vi "Calibration_user_input.vi"(4 "data mode":enum16{"Take new data point", "Refit Curve"}(ring), 6 "Mode":T5, 7 "Fixed n":bool, 8 "OK":T12, 9 "Sampling speeds":T6={"Samples /ch"=300, "Sampling Rate /ch (Hz)"=50.0} {"Sampling Rate /ch (Hz)" min=0 format="%.2f"; "Samples /ch" min=0 step=1}) -> (0 "Ch & Spans":T1[](array[typedef]) {"Ch No" min=0 max=7; "low limit (-10V)" min=-10 max=10 format="%.3f"; "high limit (10V)" min=-10 max=10 format="%.3f"}, 1 "Sampling speeds Output":T6={"Samples /ch"=300, "Sampling Rate /ch (Hz)"=50.0} {"Sampling Rate /ch (Hz)" min=0 format="%.2f"; "Samples /ch" min=0 step=1}, 2 "Fixed n out":bool, 3 "Temp (deg C)":dbl=21.0 format="%.1f", 5 "Abs Press (mbar)":dbl=1013.0 format="%.1f")   [LabVIEW 2013]
uses:
  Globals/Calib_global.vi
  Globals/Meas_global.vi
  Controls/Ref_Inst_type.ctl
  Controls/Setup.ctl
  Globals/LDA_meas_global_2.vi
  ADAM Client/Sub VIs/ADAM Controls/Channel_names.ctl
  Calib_mode.ctl
  Controls/Cal_Inst_type.ctl
  Controls/Inst_type.ctl
  Controls/PWA_Data.ctl
  Controls/ok_button.ctl
  Globals/LDA_meas_global_1.vi
  File/Setup_Filetype.ctl
  Controls/LDA_Setup.ctl
  Calib_setup.ctl
  Controls/Calibration.ctl
  Controls/TypeCalib.ctl
panel:
  in  "Acquisition Plug in":u16(ring) items=["ADAM_Server_Channels.vi", "Channels_and_Index.ctl", "DataTranslation.vi", "DT_With_Multiplexer.vi", "LDA_IP.vi", "NI-DAQmx.vi", "Simulate_kernal.vi"]
  in  "PWA Data":T2
  in  "Preston tube diammeter in mm":dbl min=0.0
  in  "Reference instrument Orig":T4={"high limit (10V)"=4.0, "low limit (-10V)"=0.0, "Ch No"=4, "Off ch no"=0, "Calib filename"=path "", "Ref Instrument type"=enum."Enter Value"} {"Off ch no" min=0 max=1; "Ch No" min=0 max=7; "low limit (-10V)" min=-10 max=10 format="%.1f"; "high limit (10V)" min=-10 max=10 format="%.1f"}
  out "Message":string
  in  "Ref Instrument type":T3
  out "Info":string
  out "XW Angle Calib Present?":bool
  out "XW Velocity Calib Present?":bool
  in  "Edit temp and Press":bool
  out "2nd ref instrument":T7={"2nd Ref type"=enum."LDA", "2nd inst present"=TRUE}
  in  "Ref vel for angle calib":T8={"high limit (10V)"=6.0, "low limit (-10V)"=0.0, "Ch No"=4, "Off ch no"=0, "Calib filename"=path "", "Ref Instrument type"=enum."LDA"} {"Off ch no" min=0 max=1; "Ch No" min=0 max=50; "low limit (-10V)" min=-10 max=10 format="%.1f"; "high limit (10V)" min=-10 max=10 format="%.1f"}
  out "Instrument type":T9=enum."Cross wire angle"
  in  "angle calib":T10(ring)
  in  "Reference instrument":T8={"high limit (10V)"=4.0, "low limit (-10V)"=0.0, "Ch No"=4, "Off ch no"=0, "Calib filename"=path "", "Ref Instrument type"=enum."Enter Value"} {"Off ch no" min=0 max=1; "Ch No" min=0 max=50; "low limit (-10V)" min=-10 max=10 format="%.1f"; "high limit (10V)" min=-10 max=10 format="%.1f"}
  in  "instrument to calibrate":T11=[{"high limit (10V)"=5.0, "low limit (-10V)"=3.0, "Ch No"=1, "Off ch no"=1, "DAQmx Channel"=""}, {"high limit (10V)"=5.0, "low limit (-10V)"=3.0, "Ch No"=2, "Off ch no"=1, "DAQmx Channel"=""}] {"Off ch no" min=0 max=1; "Ch No" min=0 max=1000; "low limit (-10V)" min=-10 max=10 format="%.3f"; "high limit (10V)" min=-10 max=10 format="%.3f"}
  in  "Instrument type":T9=enum."Pressure Transducer"
  out "Calib filename":path
  in  "Type":T1={"high limit (10V)"=4.0, "low limit (-10V)"=0.0, "Ch No"=4, "Var name"="LDA", "DAQmx Chan"=""} {"Ch No" min=0 max=7; "low limit (-10V)" min=-10 max=10 format="%.3f"; "high limit (10V)" min=-10 max=10 format="%.3f"}
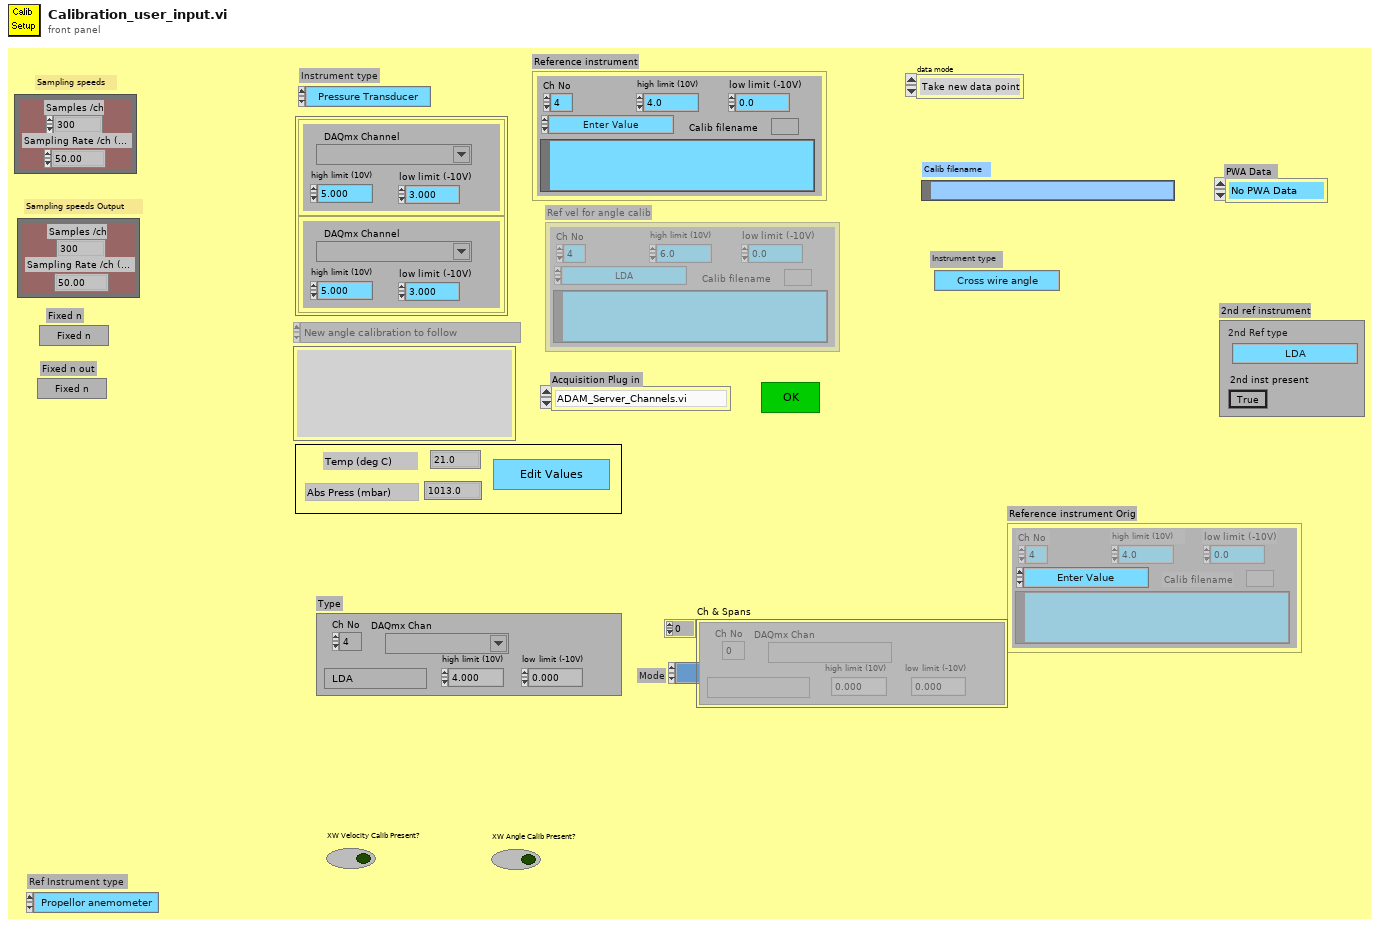
[diagram p1: front panel]
types:
  T1 = typedef "TypeCalib.ctl" = cluster{"high limit (10V)":sgl, "low limit (-10V)":sgl, "Ch No":i16, "Var name":string, "DAQmx Chan":tag}
  T2 = typedef "PWA_Data.ctl" = enum16{"No PWA Data", "One Ch PWA"}
  T3 = typedef "Ref_Inst_type.ctl" = enum16{"Propellor anemometer", "Pressure Transducer", "Raw voltage", "Pitot-static tube", "Preston tube", "Generic Linear", "Generic Polynomial", "Thermocouple", "LDA", "Enter Value", "ADAM Channel"}
  T4 = cluster{"high limit (10V)":sgl, "low limit (-10V)":sgl, "Ch No":i16, "Off ch no":i8, "Calib filename":path, "Ref Instrument type":T3}
  T5 = typedef "Calib_mode.ctl" = enum16{"Show Setup", "Take a New Calibration Point", "Refit Curve", "Setup Front Panel"}
  T6 = cluster{"Samples /ch":i32, "Sampling Rate /ch (Hz)":sgl}
  T7 = cluster{"2nd Ref type":T3, "2nd inst present":bool}
  T8 = typedef "Calib_setup.ctl" = cluster{"high limit (10V)":sgl, "low limit (-10V)":sgl, "Ch No":i16, "Off ch no":i8, "Calib filename":path, "Ref Instrument type":T3}
  T9 = typedef "Cal_Inst_type.ctl" = enum16{"Propeller anemometer", "Pressure Transducer", "Hot wire", "Cross wire velocity", "Cross wire angle", "Generic Linear", "Generic Polynomial", "Generic BackPoly", "Fast FID", "Thermocouple", "Cold wire", "Pulsed Wire"}
  T10 = enum16{"New angle calibration to follow", "Use the most recent angle calibration"}
  T11 = typedef "Calibration.ctl" = cluster{"high limit (10V)":sgl, "low limit (-10V)":sgl, "Ch No":i16, "Off ch no":i8, "DAQmx Channel":tag}[]
  T12 = typedef "ok_button.ctl" = bool
  T13 = typedef "Setup_Filetype.ctl" = enum16{"Measurement Setups", "Calibration Setups", "General", "Results File Plotter Setups", "Speed Calib Tweaks"}
  T14 = typedef "Inst_type.ctl" = enum16{"Propeller anemometer", "Raw voltage", "Pressure Transducer", "Pitot-static tube", "Preston tube", "Hot wire", "Cross wire 1", "Cross wire 2", "Generic Linear", "Generic Polynomial", "Generic BackPoly", "Fast FID", "Thermocouple", "Cold wire", "Pulsed Wire", "LDA Vel", "LDA Tran time", "LDA Arr time"}
  T15 = typedef "Channel_names.ctl" = enum16{"Active Only", "Active + Off", "All Channels"}
  T16 = typedef "LDA_Setup.ctl" = cluster{"dimensions":enum16{"1D", "2D"}, "Analogue Freq Multiplier":dbl}
  T17 = typedef "Setup.ctl" = enum16{"Run Program", "Show Setup", "Save Current Setup", "Setup Front Panel"}
  T18 = cluster{"high limit (10V)":sgl, "low limit (-10V)":sgl, "Ch No":i16, "Off ch no":i8, "DAQmx Channel":tag}
  T19 = typedef "BSA_Type.ctl" = enum16{"57N11", "BSA F60"}
  T20 = typedef "BSA_info_Cluster.ctl" = cluster{"GPIB Address":string, "No of Check Bytes":i32, "Extra Info":string, "COLOUR":u32, "Wavelength (nm)":dbl}
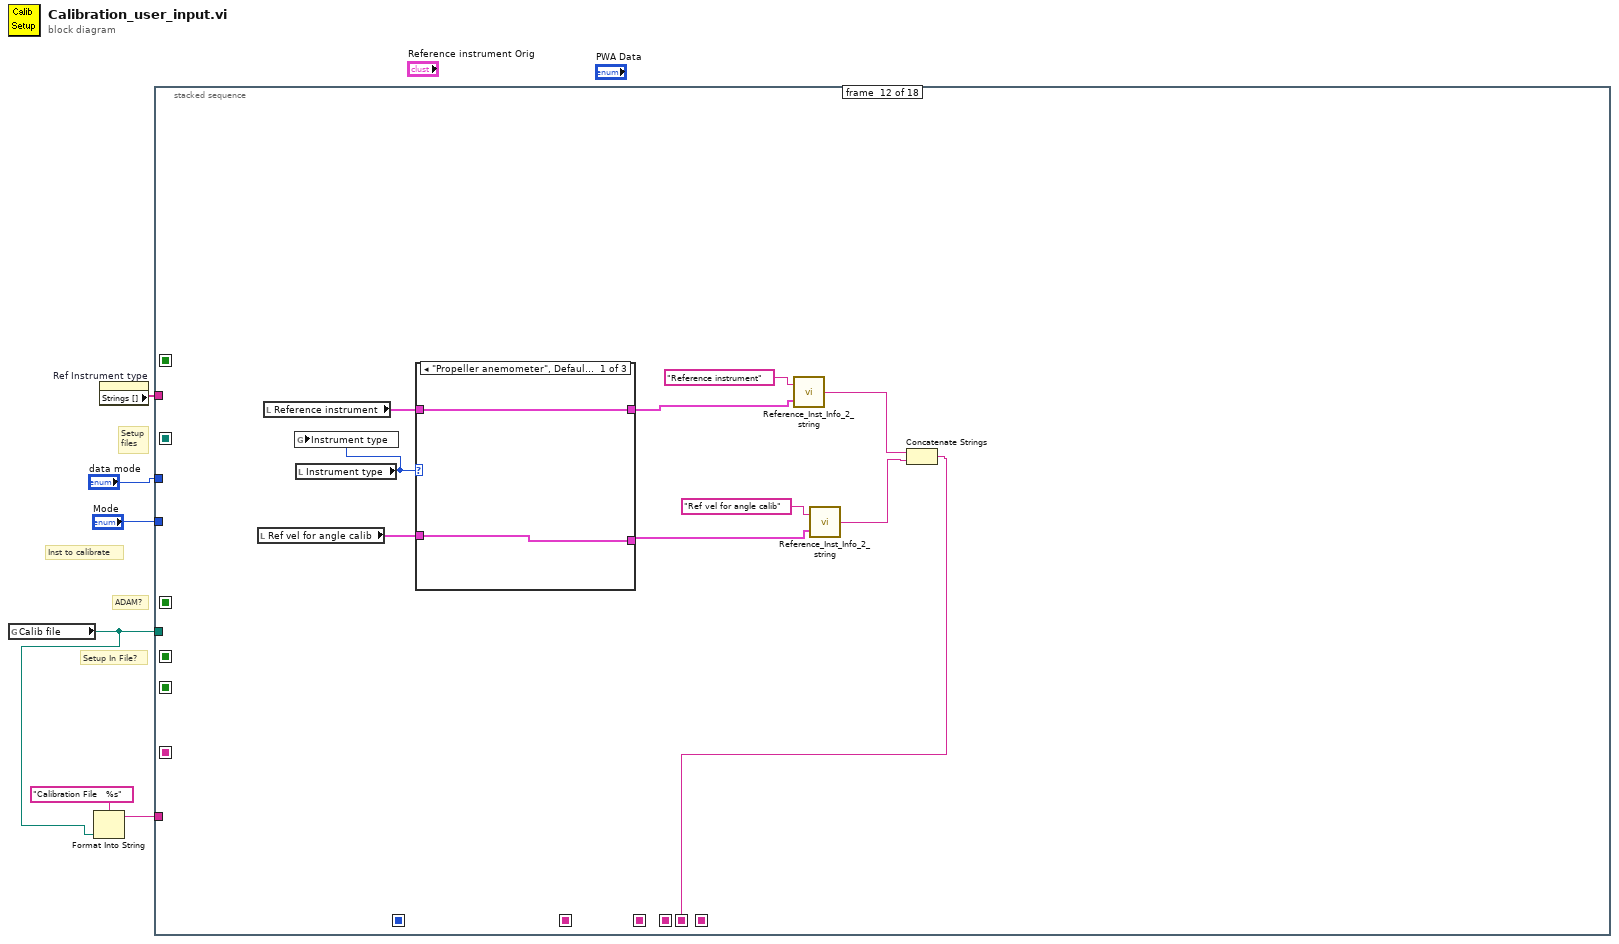
[diagram p0: block diagram]
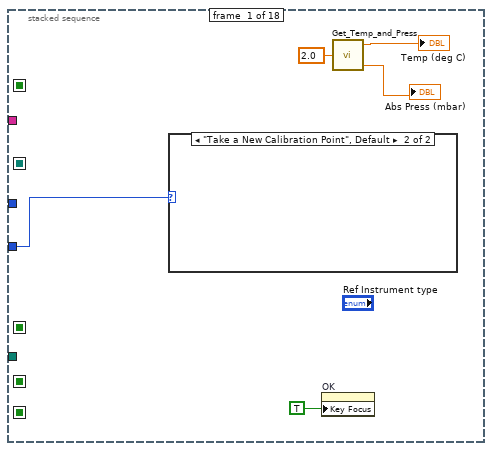
[diagram p2: hidden frame]
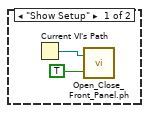
[diagram p3: hidden frame]
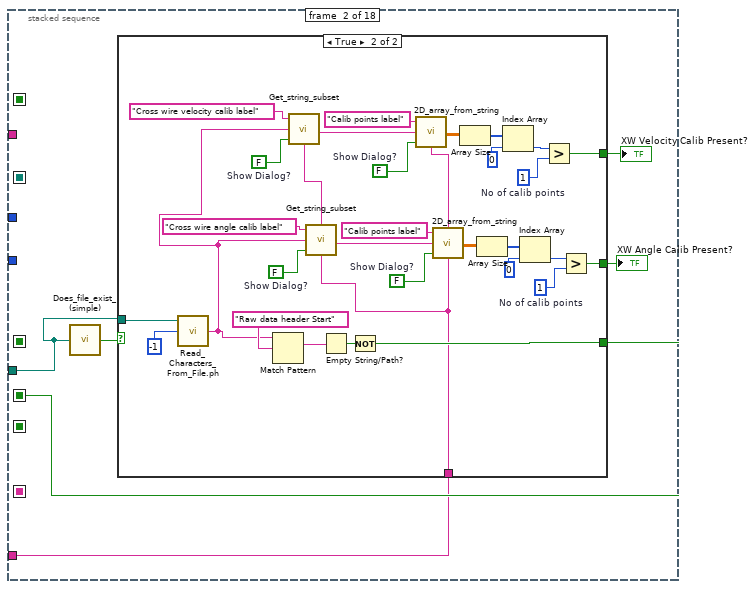
[diagram p4: hidden frame]
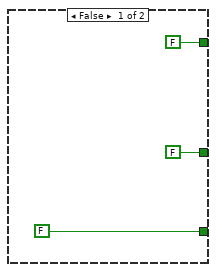
[diagram p5: hidden frame]
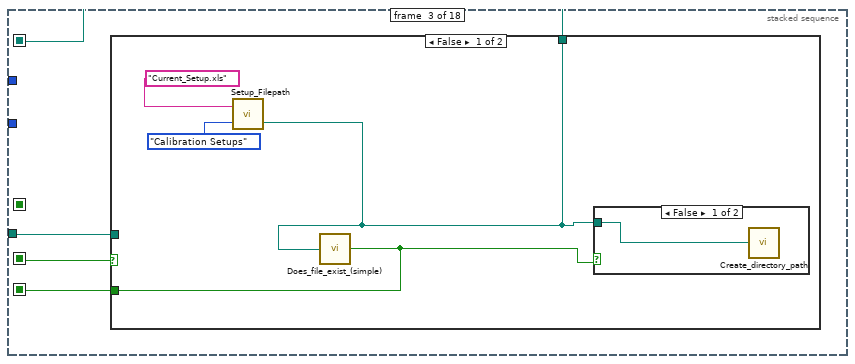
[diagram p6: hidden frame]
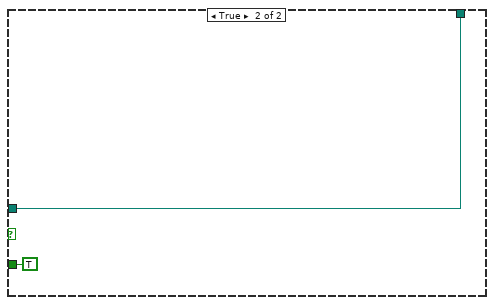
[diagram p8: hidden frame]
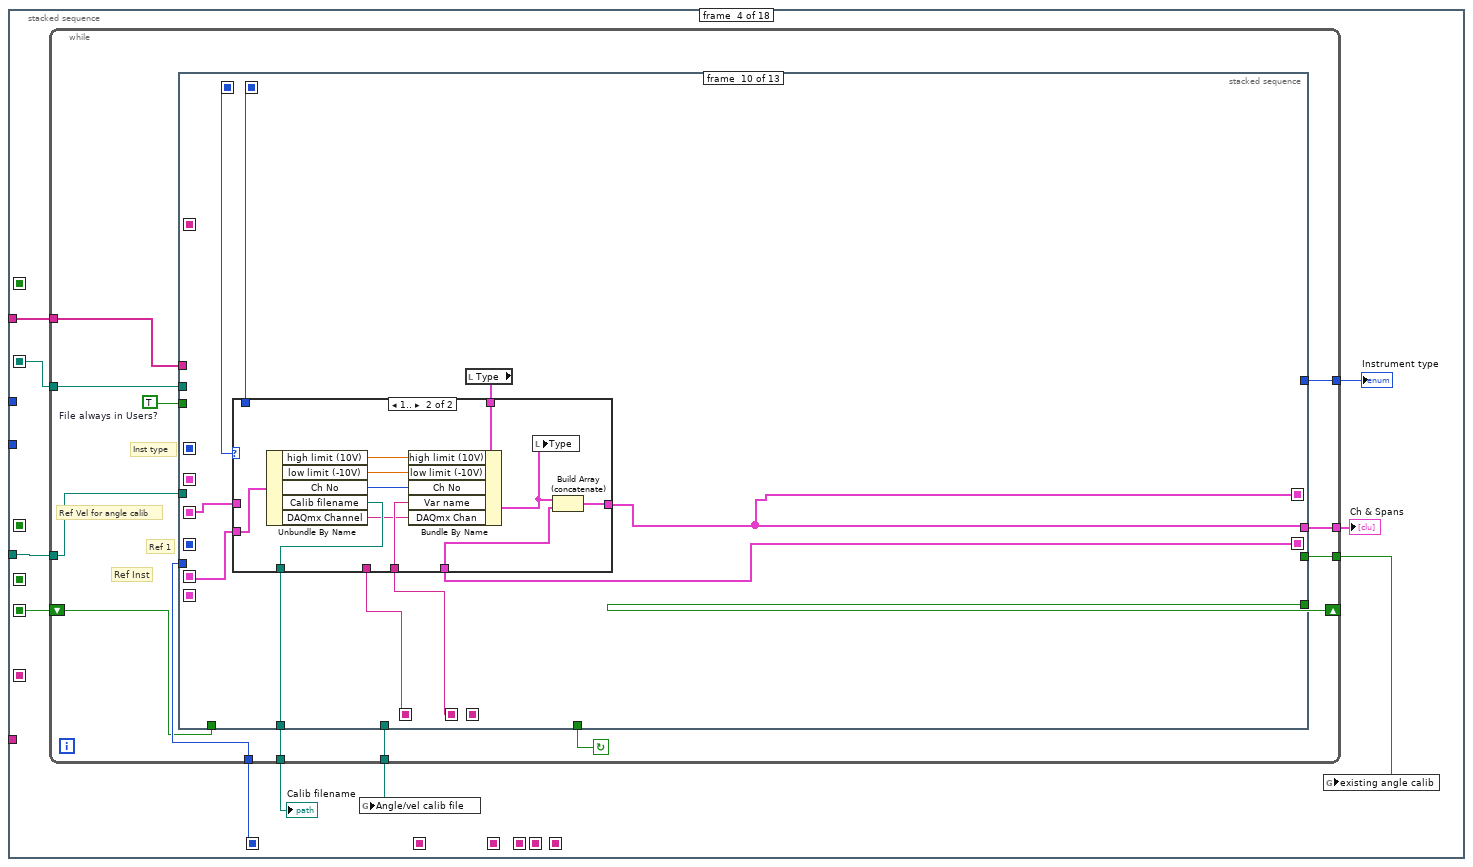
[diagram p9: hidden frame]
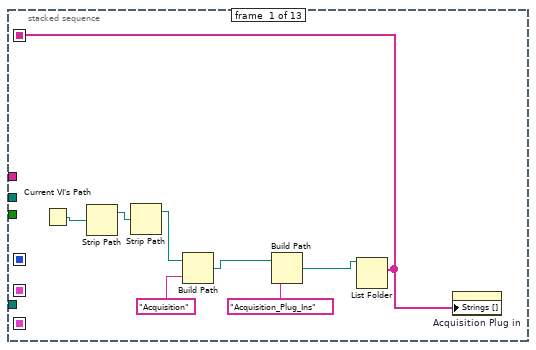
[diagram p10: hidden frame]
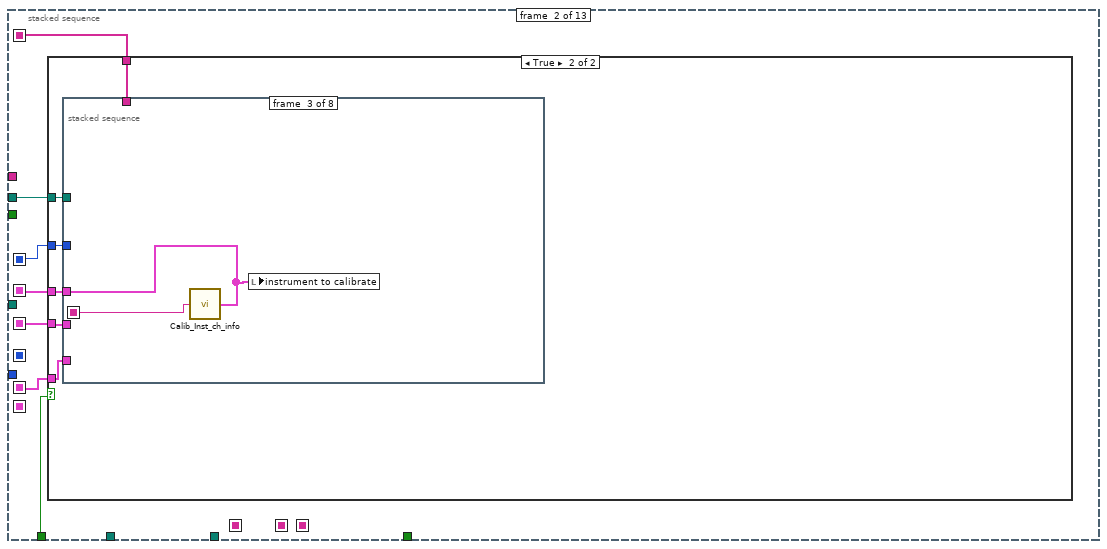
[diagram p11: hidden frame]
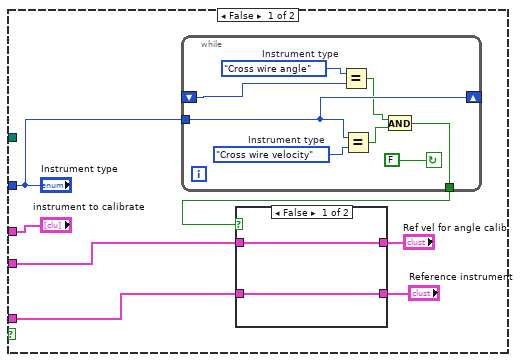
[diagram p12: hidden frame]
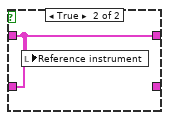
[diagram p13: hidden frame]
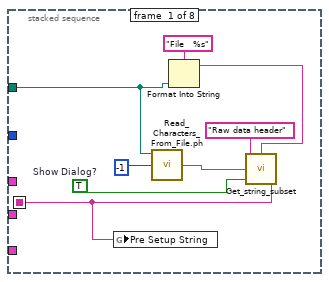
[diagram p14: hidden frame]
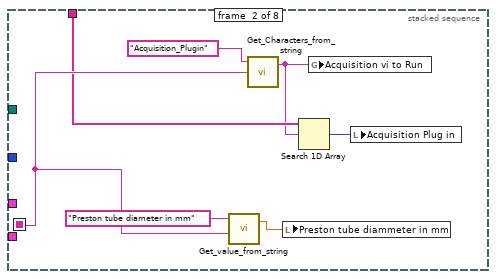
[diagram p15: hidden frame]
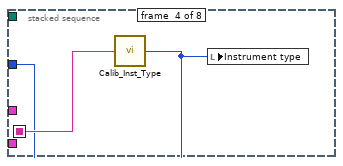
[diagram p16: hidden frame]
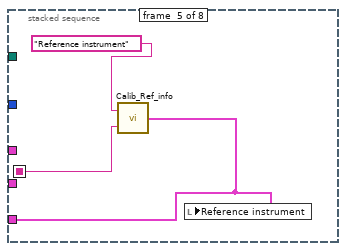
[diagram p17: hidden frame]
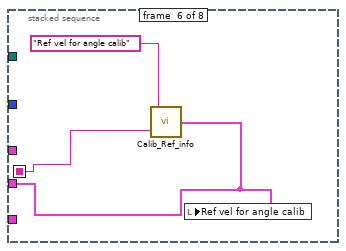
[diagram p18: hidden frame]
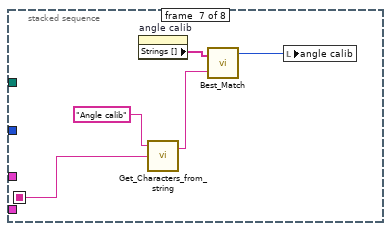
[diagram p19: hidden frame]
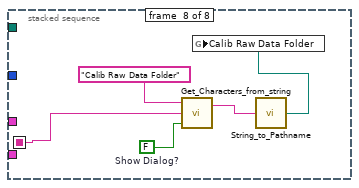
[diagram p20: hidden frame]
diagram:
  # "Inst to calibrate"
  # "Setup In File?"
  # "Setup\nfiles"
  # "ADAM?"
  n1 = global read "Calib_global.vi" "Calib file"() -> (w2:path)
  n2 = Format Into String(format string="Calibration File   %s", w2) -> (resulting string=w1:string)  [unwired: 2 in, 1 out]
  n3 = property on="Ref Instrument type" class="Enum (strict)"() -> ("Strings []"=w4:string[])  [unwired: 2 in, 2 out]
  n4 = stacked-sequence {
    seq-local: [_ _ w55 _ _ _ _ _ _ _ _ _ _ _ _ _ _ _] -> [_ _ _ w72 _ _ _ _ _ _ _ _ _ _ _ _ _ _]
    seq-local: [_ _ w56 _ _ _ _ _ _ _ _ _ _ _ _ _ _ _] -> [_ _ _ w70 _ _ _ _ _ _ _ _ _ _ _ _ _ _]
    seq-local: [_ _ _ w69 _ _ _ _ _ _ _ _ _ _ _ _ _ _] -> [_ _ _ _ _ _ _ w623 _ _ _ _ _ _ _ _ _ _]
    seq-local: [_ _ _ _ _ _ _ w624 _ _ _ _ _ _ _ _ _ _] -> [_ _ _ _ _ _ _ _ w641 _ _ _ _ _ _ _ _ _]
    seq-local: [_ _ _ _ _ _ _ _ w644 _ _ _ _ _ _ _ _ _] -> [_ _ _ _ _ _ _ _ _ _ _ _ _ _ w831 _ _ _]
    seq-local: [_ _ _ _ _ _ _ _ _ _ w733 _ _ _ _ _ _ _] -> [_ _ _ _ _ _ _ _ _ _ _ _ _ _ w830 _ w868 _]
    seq-local: [_ _ _ _ _ _ _ _ _ _ w730 _ _ _ _ _ _ _] -> [_ _ _ _ _ _ _ _ _ _ _ _ _ _ _ w837 _ _]
    seq-local: [_ w19 _ _ _ _ _ _ _ _ _ _ _ _ _ _ _ _] -> [_ _ w54 _ _ _ _ _ _ _ _ _ _ _ _ _ _ _]
    seq-local: [_ _ _ _ _ _ _ _ _ _ _ w745 _ _ _ _ _ _] -> [_ _ _ _ _ _ _ _ _ _ _ _ _ _ w823 _ _ _]
    seq-local: [_ _ _ _ _ _ _ _ _ _ _ _ _ w773 _ _ _ _] -> [_ _ _ _ _ _ _ _ _ _ _ _ _ _ w811 _ _ _]
    seq-local: [_ _ _ _ _ _ _ _ _ _ _ _ w752 _ _ _ _ _] -> [_ _ _ _ _ _ _ _ _ _ _ _ _ _ w807 _ w859 _]
    seq-local: [_ _ _ _ _ _ _ _ _ w679 _ _ _ _ _ _ _ _] -> [_ _ _ _ _ _ _ _ _ _ _ _ _ _ w806 _ _ _]
    tunnel: "Mode" -> [w7 _ _ _ w546 w564 _ _ w643 w692 _ _ w753 _ _ w839 _ w885]
    tunnel: "data mode" -> [_ _ _ _ w540 _ _ _ _ _ _ _ _ _ _ _ _ _]
    tunnel: w2 -> [_ w17 w53 w66 _ _ _ _ _ _ _ _ _ _ _ _ _ _]
    tunnel: w4 -> [_ _ _ w65 _ _ _ _ _ _ _ _ _ _ _ _ _ _]
    tunnel: w1 -> [_ w14 _ _ _ _ _ _ _ _ _ _ _ _ _ _ _ _]
    frame #0 {
      n5 = case shown="\"Take a New Calibration Point\", Default" w7 {
        frame "Show Setup" {
          n6 = Current VI's Path() -> (path=w13:path)
          n7 = call "Open_Close_Front_Panel.ph.vi"("Front Panel Window:Open"=TRUE, "VI path"=w13) -> ()  [unwired: 2 out]
        }
        frame "Take a New Calibration Point", Default {
        }
      }
      n8 = property on="OK" class="Bool"("Key Focus"=TRUE) -> ()  [unwired: 2 in, 2 out]
      n9 = call "Get_Temp_and_Press.vi"("Averaging time (mins)"=2.0) -> ("Abs Press (mbar)"=→"Abs Press (mbar)":dbl, "Temperature"=→"Temp (deg C)":dbl)  [unwired: 3 out]
    }
    frame #1 {
      n10 = call "Does_file_exist_(simple).vi"("Pathname"=w17) -> ("exists?"=w18:bool)
      n11 = case shown="True" w18 {
        tunnel: [FALSE w48] -> w19
        tunnel: w17 -> [_ w47]
        tunnel: [FALSE w25] -> w16
        tunnel: [FALSE w24] -> w15
        tunnel: w14 -> [_ w23]
        frame False {
        }
        frame True {
          w36 = 1  # No of calib points
          w30 = FALSE  # Show Dialog?
          w28 = FALSE  # Show Dialog?
          w37 = 1  # No of calib points
          w43 = FALSE  # Show Dialog?
          w45 = FALSE  # Show Dialog?
          n12 = call "Read_Characters_From_File.ph.vi"("file path (dialog if empty)"=w47, "number of characters (all:-1)"=-1) -> ("character string"=w26:string)  [unwired: 7 out]
          n13 = Match Pattern(string=w26, regular expression="Raw data header Start") -> (match substring=w50:string)  [unwired: 4 out]
          n14 = call "Get_string_subset.vi"("String Name"=w23, "Show Dialog?"=w28, "String to split"=w26, "File Label"="Cross wire velocity calib label") -> ("Output string"=w34:string)  [unwired: 1 out]
          n15 = call "Get_string_subset.vi"("String Name"=w23, "Show Dialog?"=w45, "String to split"=w26, "File Label"="Cross wire angle calib label") -> ("Output string"=w39:string)  [unwired: 1 out]
          n16 = Empty String/Path?(string/path=w50) -> (empty?=w49:bool)
          n17 = Not(x=w49) -> (.not. x?=w48:bool)
          n18 = call "2D_array_from_string.vi"("String Name"=w23, "Show Dialog?"=w30, "Input string"=w34, "Array title"="Calib points label") -> ("2D data array"=w31:dbl[][])
          n19 = call "2D_array_from_string.vi"("String Name"=w23, "Show Dialog?"=w43, "Input string"=w39, "Array title"="Calib points label") -> ("2D data array"=w42:dbl[][])
          n20 = Array Size(array=w31) -> (size(s)=w32:i32[])
          n21 = Array Size(array=w42) -> (size(s)=w41:i32[])
          n22 = Index Array(array=w32, index=0 ("Index")) -> (element=w35:i32)
          n23 = Index Array(array=w41, index=0 ("Index")) -> (element=w38:i32)
          n24 = Greater?(x=w35, y=w36) -> (0:w24:bool)
          n25 = Greater?(x=w38, y=w37) -> (0:w25:bool)
        }
      }
      "XW Velocity Calib Present?" <- w15
      "XW Angle Calib Present?" <- w16
    }
    frame #2 {
      n26 = case shown="False" w54 {
        tunnel: [w60 TRUE ("exists")] -> w56
        tunnel: [w57 w63] -> w55
        tunnel: w53 -> [_ w63]
        frame False {
          n27 = call "Setup_Filepath.vi"("Setup File Type"=Setup_Filetype."Calibration Setups", "Filename in"="Current_Setup.xls") -> ("Filename Out"=w57:path)  [unwired: 1 out]
          n28 = call "Does_file_exist_(simple).vi"("Pathname"=w57) -> ("exists?"=w60:bool)
          n29 = case shown="False" w60 {
            tunnel: w57 -> [w61 _]
            frame False {
              n30 = call "Create_directory_path.vi"("Path name"=w61) -> ()  [unwired: 1 in, 2 out]
            }
            frame True {
            }
          }
        }
        frame True {
        }
      }
    }
    frame #3 {
      n31 = while {
        tunnel: w65 -> [w77]
        shift-left: w70 -> [w80]
        shift-right: [w79] -> _
        tunnel: [w81] -> w71
        tunnel: w72 -> [w82]
        tunnel: [w83] -> w68
        tunnel: [w84] -> w64
        tunnel: [w85] -> w69
        tunnel: [w86] -> w73
        tunnel: [w75] -> w67
        tunnel: w66 -> [w74]
        stop <- w78 continue-if-true
        w76 = TRUE  # File always in Users?
        # "Ref 1"
        # "Ref Inst"
        # "Ref Vel for angle calib"
        # "Inst type"
        n32 = stacked-sequence {
          seq-local: [_ _ w166 _ _ _ _ _ _ _ _ _ _] -> [_ _ _ _ _ w290 _ _ _ _ _ _ _]
          seq-local: [_ _ w170 _ _ _ _ _ _ _ _ _ _] -> [_ _ _ _ _ _ _ _ w441 _ _ _ _]
          seq-local: [_ _ _ _ _ w284 _ _ _ _ _ _ _] -> [_ _ _ _ _ _ _ _ _ w459 _ _ _]
          seq-local: [_ _ w165 _ _ _ _ _ _ _ _ _ _] -> [_ _ _ _ _ _ _ _ _ w457 _ _ _]
          seq-local: [_ _ _ _ _ _ _ _ w440 _ _ _ _] -> [_ _ _ _ _ _ _ _ _ w458 _ _ _]
          seq-local: [_ _ _ _ _ _ _ w362 _ _ _ _ _] -> [_ _ _ _ _ _ _ _ _ w454 _ _ _]
          seq-local: [_ _ _ _ _ _ w358 _ _ _ _ _ _] -> [_ _ _ _ _ _ _ _ _ w453 _ _ _]
          seq-local: [_ w99 _ _ _ _ _ _ _ _ _ _ _] -> [_ _ w168 w201 w214 _ _ w363 _ _ _ _ _]
          seq-local: [_ w98 _ _ _ _ _ _ _ _ _ _ _] -> [_ _ _ w200 _ _ _ _ _ _ _ _ _]
          seq-local: [_ w97 _ _ _ _ _ _ _ _ _ _ _] -> [_ _ _ _ _ _ w360 w364 _ w452 _ _ _]
          seq-local: [_ w96 _ _ _ _ _ _ _ _ _ _ _] -> [_ _ w167 _ _ _ _ _ _ w451 _ _ w539]
          seq-local: [_ _ _ _ _ _ _ _ _ w450 _ _ _] -> [_ _ _ _ _ _ _ _ _ _ _ w498 _]
          seq-local: [_ _ _ w196 _ _ _ _ _ _ _ _ _] -> [_ _ _ _ _ _ _ _ w439 _ _ _ _]
          seq-local: [w87 _ _ _ _ _ _ _ _ _ _ _ _] -> [_ w95 _ _ _ _ _ _ _ _ _ _ _]
          tunnel: [_ _ _ _ _ _ _ _ _ w456 _ _ _] -> w86
          tunnel: [_ _ w166 _ _ _ _ _ _ _ _ _ _] -> w85
          tunnel: [_ _ _ _ _ _ _ _ _ w450 _ _ _] -> w84
          tunnel: [_ _ _ _ w219 _ _ _ _ _ _ _ _] -> w83
          tunnel: w82 -> [_ w101 _ _ _ _ _ _ _ _ _ _ _]
          tunnel: [_ _ w168 _ _ _ _ _ _ _ _ _ _] -> w81
          tunnel: w80 -> [_ w100 _ _ _ _ _ _ _ _ _ _ _]
          tunnel: [_ _ _ _ _ _ _ _ _ _ _ FALSE _] -> w79
          tunnel: [_ _ _ _ _ _ _ _ _ _ _ w496 _] -> w78
          tunnel: w77 -> [_ _ w164 _ _ _ w357 _ _ _ _ _ _]
          tunnel: w76 -> [_ _ _ _ _ _ _ _ _ _ _ _ _]
          tunnel: [_ _ _ _ w218 _ _ _ _ _ _ _ _] -> w75
          tunnel: w74 -> [_ _ _ _ w220 _ _ _ _ _ _ _ _]
          frame #0 {
            n33 = Current VI's Path() -> (path=w90:path)
            n34 = Strip Path(path=w90) -> (stripped path=w89:path)  [unwired: 1 out]
            n35 = Strip Path(path=w89) -> (stripped path=w88:path)  [unwired: 1 out]
            n36 = Build Path(base path=w88, name or relative path="Acquisition") -> (appended path=w93:path)
            n37 = Build Path(base path=w93, name or relative path="Acquisition_Plug_Ins") -> (appended path=w94:path)
            n38 = List Folder(path=w94) -> (filenames=w87:string[])  [unwired: 3 in, 3 out]
            n39 = property on="Acquisition Plug in" class="Ring (strict)"("Strings []"=w87) -> ()  [unwired: 2 in, 2 out]
          }
          frame #1 {
            n40 = case shown="True" w100 {
              tunnel: w101 -> [_ w125]
              tunnel: ["Instrument type" w123] -> w99
              tunnel: ["instrument to calibrate" w124] -> w98
              tunnel: [w103 w121] -> w97
              tunnel: [w105 w122] -> w96
              tunnel: w95 -> [_ w120]
              frame False {
                n41 = while {
                  shift-right: [w117] -> _
                  shift-left: _ -> [w115]
                  tunnel: "Instrument type" -> [w117]
                  tunnel: [w112] -> w106
                  stop <- FALSE continue-if-true
                  w116 = Cal_Inst_type."Cross wire angle"  # Instrument type
                  w118 = Cal_Inst_type."Cross wire velocity"  # Instrument type
                  n42 = Equal?(x=w116, y=w115) -> (x = y?=w113:bool)
                  n43 = Equal?(x=w117, y=w118) -> (x = y?=w114:bool)
                  n44 = And(x=w113, y=w114) -> (x .and. y?=w112:bool)
                }
                n45 = case shown="False" w106 {
                  tunnel: [w110 w111] -> w105
                  tunnel: "Reference instrument" -> [w110 _]
                  tunnel: [w109 w111] -> w103
                  tunnel: "Ref vel for angle calib" -> [w109 w111]
                  frame False {
                  }
                  frame True {
                    n46 = local write "Reference instrument"(w111) -> ()
                  }
                }
              }
              frame True {
                n47 = stacked-sequence {
                  seq-local: [w130 _ _ _ _ _ _ _] -> [_ w137 w142 w144 w146 w149 w153 w158]
                  tunnel: w125 -> [w127 _ _ _ _ _ _ _]
                  tunnel: [_ _ w141 _ _ _ _ _] -> w124
                  tunnel: [_ _ _ w143 _ _ _ _] -> w123
                  tunnel: [_ _ _ _ w145 _ _ _] -> w122
                  tunnel: [_ _ _ _ _ w148 _ _] -> w121
                  tunnel: w120 -> [_ w136 _ _ _ _ _ _]
                  frame #0 {
                    w129 = TRUE  # Show Dialog?
                    n48 = call "Read_Characters_From_File.ph.vi"("file path (dialog if empty)"=w127, "number of characters (all:-1)"=-1) -> ("character string"=w133:string)  [unwired: 7 out]
                    n49 = Format Into String(format string="File   %s", w127) -> (resulting string=w126:string)  [unwired: 2 in, 1 out]
                    n50 = call "Get_string_subset.vi"("String Name"=w126, "Show Dialog?"=w129, "String to split"=w133, "File Label"="Raw data header") -> ("Output string"=w130:string)  [unwired: 1 out]
                    n51 = global write "Calib_global.vi" "Pre Setup String"(w130) -> ()
                  }
                  frame #1 {
                    n52 = call "Get_value_from_string.vi"("Input string"=w137, "Variable name"="Preston tube diameter in mm") -> ("Value"=w139:dbl)  [unwired: 1 in, 1 out]
                    n53 = call "Get_Characters_from_string.vi"("Input string"=w137, "Variable name"="Acquisition_Plugin") -> ("Value"=w135:string)  [unwired: 1 in, 1 out]
                    n54 = local write "Preston tube diammeter in mm"(w139) -> ()
                    n55 = Search 1D Array(1D array=w136, element=w135) -> (index of element=w134:i32)  [unwired: 1 out]
                    n56 = global write "Meas_global.vi" "Acquisition vi to Run"(w135) -> ()
                    n57 = local write "Acquisition Plug in"(w134) -> ()
                  }
                  frame #2 {
                    n58 = call "Calib_Inst_ch_info.vi"("Input string"=w142) -> ("instrument to calibrate (new)"=w141:T11)
                    n59 = local write "instrument to calibrate"(w141) -> ()
                  }
                  frame #3 {
                    n60 = call "Calib_Inst_Type.vi"("Input string"=w144) -> ("Instrument type"=w143:T9)
                    n61 = local write "Instrument type"(w143) -> ()
                  }
                  frame #4 {
                    n62 = call "Calib_Ref_info.vi"("Input string"=w146, "Reference Name"="Reference instrument") -> ("Reference instrument"=w145:T8)
                    n63 = local write "Reference instrument"(w145) -> ()
                  }
                  frame #5 {
                    n64 = call "Calib_Ref_info.vi"("Input string"=w149, "Reference Name"="Ref vel for angle calib") -> ("Reference instrument"=w148:T8)
                    n65 = local write "Ref vel for angle calib"(w148) -> ()
                  }
                  frame #6 {
                    n66 = property on="angle calib" class="Enum (strict)"() -> ("Strings []"=w155:string[])  [unwired: 2 in, 2 out]
                    n67 = call "Get_Characters_from_string.vi"("Input string"=w153, "Variable name"="Angle calib") -> ("Value"=w152:string)  [unwired: 1 in, 1 out]
                    n68 = call "Best_Match.vi"("Input String"=w152, "String Options"=w155) -> ("index of element"=w151:i32)  [unwired: 1 out]
                    n69 = local write "angle calib"(w151) -> ()
                  }
                  frame #7 {
                    w159 = FALSE  # Show Dialog?
                    n70 = call "Get_Characters_from_string.vi"("Show Dialog?"=w159, "Input string"=w158, "Variable name"="Calib Raw Data Folder") -> ("Value"=w157:string)  [unwired: 1 out]
                    n71 = call "String_to_Pathname.vi"("Input String"=w157) -> ("path"=w156:path)
                    n72 = global write "Calib_global.vi" "Calib Raw Data Folder"(w156) -> ()
                  }
                }
              }
            }
          }
          frame #2 {
            # "#optimation Added 11/1/13"
            n73 = Unbundle By Name(w167) -> ("Ref Instrument type"=w169:T3)
            n74 = case shown="\"Cross wire angle\"" w168 {
              tunnel: [w181 w189 w194] -> w170
              tunnel: w169 -> [w179 w183 w193]
              tunnel: [w179 w186 w193] -> w166
              tunnel: w167 -> [_ w187 _]
              frame "Cross wire velocity" {
                n75 = Build Array("Raw voltage", "Raw voltage") -> (w181:string[])
              }
              frame "Cross wire angle" {
                n76 = case shown="\"ADAM Channel\"" w183 {
                  tunnel: [w190 w191 Ref_Inst_type."Enter Value" ("Ref Instrument type")] -> w186
                  tunnel: w183 -> [w190 w191 _]
                  frame "Enter Value" {
                  }
                  frame "ADAM Channel" {
                  }
                  frame "LDA", Default {
                  }
                }
                n77 = Bundle By Name(cluster=w187, "Ref Instrument type"=w186) -> (w188:T8)
                n78 = local write "Reference instrument"(w188) -> ()
                n79 = Build Array("Raw voltage", "Raw voltage") -> (w189:string[])
              }
              frame "Generic Linear", Default {
                n80 = Build Array("Raw voltage") -> (w194:string[])
              }
            }
            n81 = Index Array(array=w164, index=w166) -> (element=w165:string)
            n82 = property on="Acquisition Plug in" class="Ring (strict)"() -> ("Strings []"=w163:string[])  [unwired: 2 in, 2 out]
            n83 = Index Array(array=w163, index="Acquisition Plug in") -> (element=w161:string)
            n84 = case shown="\"NI-DAQmx.vi\"" w161 {
              frame "False", Default {
                (unwired) FALSE ("Visible")
                (unwired) FALSE ("Visible")
                n85 = property on="DAQmx Channel" class="DAQmxName"("Visible"=FALSE) -> ()  [unwired: 2 in, 2 out]
                n86 = property on="Ch No" class="DigNum (strict)"("Visible"=TRUE) -> ()  [unwired: 2 in, 2 out]
                n87 = property on="Ch No" class="DigNum (strict)"("Visible"=TRUE) -> ()  [unwired: 2 in, 2 out]
                n88 = property on="Ch No" class="DigNum (strict)"("Visible"=TRUE) -> ()  [unwired: 2 in, 2 out]
              }
              frame "NI-DAQmx.vi" {
                (unwired) TRUE ("Visible")
                (unwired) TRUE ("Visible")
                n89 = property on="DAQmx Channel" class="DAQmxName"("Visible"=TRUE) -> ()  [unwired: 2 in, 2 out]
                n90 = property on="Ch No" class="DigNum (strict)"("Visible"=FALSE) -> ()  [unwired: 2 in, 2 out]
                n91 = property on="Ch No" class="DigNum (strict)"("Visible"=FALSE) -> ()  [unwired: 2 in, 2 out]
                n92 = property on="Ch No" class="DigNum (strict)"("Visible"=FALSE) -> ()  [unwired: 2 in, 2 out]
              }
            }
            n93 = global write "Meas_global.vi" "Acquisition vi to Run"(w161) -> ()
          }
          frame #3 {
            n94 = Array Size(array=w200) -> (size(s)=w199:i32)
            n95 = case shown="\"Cross wire angle\"" w201 {
              tunnel: [2 2 1 0] -> w198
              frame "Cross wire velocity" {
              }
              frame "Cross wire angle" {
              }
              frame "Generic Linear", Default {
              }
              frame "Pulsed Wire" {
              }
            }
            n96 = Equal?(x=w198, y=w199) -> (x = y?=w197:bool)
            n97 = case shown="False" w197 {
              tunnel: w198 -> [w207 _]
              tunnel: w200 -> [w203 w209]
              tunnel: [w202 w209] -> w196
              frame False {
                n98 = Index Array(array=w203, index=0) -> (element=w204:T18)
                n99 = Build Array (concatenate)(w203, w204) -> (w206:T11)
                n100 = for {
                  N: w207 -> [_]
                  tunnel: w206 -> [w208] mode=indexing
                  tunnel: [w208] -> w202 mode=indexing
                }
                n101 = local write "instrument to calibrate"(w202) -> ()
              }
              frame True {
              }
            }
          }
          frame #4 {
            n102 = case shown="\"Cross wire angle\"" w214 {
              tunnel: w220 -> [_ w231 w253]
              tunnel: [path "" w232 w254] -> w219
              tunnel: [FALSE w230 w252] -> w218
              tunnel: [w221 w226 w248] -> w217
              tunnel: [w223 w229 w251] -> w216
              tunnel: ["" w228 w249] -> w215
              tunnel: w214 -> [_ w227 w250]
              frame "Propeller anemometer", Default {
                w221 = u8 2  # Disabled
                w223 = u8 2  # Disabled
              }
              frame "Cross wire angle" {
                w226 = u8 0  # Disabled
                w229 = u8 2  # Disabled
                n103 = local read "XW Velocity Calib Present?"() -> (w233:bool)
                n104 = case shown="False" w233 {
                  tunnel: [w237 w247] -> w232
                  tunnel: w231 -> [_ w247]
                  tunnel: [TRUE TRUE] -> w230
                  tunnel: [w235 w245] -> w228
                  tunnel: w227 -> [w234 _]
                  frame False {
                    w241 = 0  # index
                    n105 = local read "instrument to calibrate"() -> (w242:T11)
                    n106 = Index Array(array=w242, index=w241) -> (element=w240:T18)
                    n107 = Unbundle By Name(w240) -> ("Ch No"=w238:i16)
                    n108 = call "XW_file_info.vi"("Instrument type"=w234, "Ch No"=w238) -> ("Filename"=w237:path, "resulting string"=w235:string, "File Exists?"=w236:bool)
                    n109 = case shown="False" w236 {
                      frame False {
                        w243 = Cal_Inst_type."Cross wire velocity"  # Instrument type
                        w244 = "You need to do a velocity calibration before you can do the angle calibration"  # message
                        n110 = local write "Instrument type"(w243) -> ()
                        n111 = One Button Dialog(message=w244) -> ()  [unwired: 2 out]
                      }
                      frame True {
                      }
                    }
                  }
                  frame True {
                    w245 = "Will use the velocity Calibration info already in the Calibration file. "  # resulting string
                  }
                }
              }
              frame "Cross wire velocity" {
                w248 = u8 2  # Disabled
                n112 = local read "XW Angle Calib Present?"() -> (w255:bool)
                n113 = case shown="False" w255 {
                  tunnel: [w264 w283] -> w254
                  tunnel: w253 -> [_ w283]
                  tunnel: [TRUE FALSE] -> _
                  tunnel: [w263 TRUE] -> w252
                  tunnel: [w262 w280] -> w251
                  tunnel: w250 -> [w260 _]
                  tunnel: [w257 w279] -> w249
                  frame False {
                    w268 = 0  # index
                    n114 = local read "instrument to calibrate"() -> (w269:T11)
                    n115 = Index Array(array=w269, index=w268) -> (element=w267:T18)
                    n116 = Unbundle By Name(w267) -> ("Ch No"=w261:i16)
                    n117 = call "XW_file_info.vi"("Instrument type"=w260, "Ch No"=w261) -> ("Filename"=w259:path, "resulting string"=w256:string, "File Exists?"=w258:bool)
                    n118 = case shown="\"New angle calibration to follow\"" "angle calib" {
                      tunnel: [path "" w275] -> w264
                      tunnel: w259 -> [_ w275]
                      tunnel: [FALSE TRUE] -> w263
                      tunnel: ["This XW velocity Calibration MUST be followed by an angle calibration, before XW measurements can be made." w273] -> w257
                      tunnel: w256 -> [_ w273]
                      frame "New angle calibration to follow" {
                      }
                      frame "Use the most recent angle calibration" {
                      }
                    }
                    n119 = case shown="False" w258 {
                      tunnel: [w276 w278] -> w262
                      frame False {
                        w276 = u8 2  # Disabled
                        w277 = T10."New angle calibration to follow"  # angle calib
                        n120 = local write "angle calib"(w277) -> ()
                      }
                      frame True {
                        w278 = u8 0  # Disabled
                      }
                    }
                  }
                  frame True {
                    w279 = "Will use the angle Calibration info already in the Calibration file. "  # resulting string
                    w280 = u8 0  # Disabled
                  }
                }
              }
            }
            "Info" <- w215
            n121 = property on="Ref vel for angle calib" class="Clust (strict)"("Disabled"=w217) -> ()  [unwired: 2 in, 2 out]
            n122 = property on="angle calib" class="Enum (strict)"("Disabled"=w216) -> ()  [unwired: 2 in, 2 out]
          }
          frame #5 {
            n123 = case shown="\"Enter Value\"" w290 {
              tunnel: [u8 0 u8 0 u8 0 u8 0 u8 0 u8 0 u8 0 u8 2 u8 2 u8 2 u8 2] -> w285
              tunnel: [u8 0 u8 0 u8 2 u8 0 u8 0 u8 0 u8 0 u8 2 u8 2 u8 2 u8 2] -> w289
              tunnel: [u8 0 u8 0 u8 0 u8 0 u8 0 u8 0 u8 0 u8 2 u8 2 u8 2 u8 2] -> w288
              tunnel: [u8 0 u8 0 u8 0 u8 0 u8 0 u8 0 u8 0 u8 2 u8 2 u8 2 u8 2] -> w287
              tunnel: [u8 0 u8 0 u8 0 u8 0 u8 0 u8 0 u8 0 u8 2 u8 2 u8 2 u8 2] -> w286
              tunnel: [1 1 1 1 1 1 1 0 0 0 0] -> w284
              frame "Propellor anemometer" {
              }
              frame "Pressure Transducer" {
              }
              frame "Raw voltage" {
              }
              frame "Pitot-static tube" {
              }
              frame "Preston tube" {
              }
              frame "Generic Linear" {
              }
              frame "Generic Polynomial" {
              }
              frame "Thermocouple" {
              }
              frame "LDA" {
              }
              frame "Enter Value" {
              }
              frame "ADAM Channel" {
              }
            }
            n124 = property on="Calib filename" class="Path"("Disabled"=w289) -> ()  [unwired: 2 in, 2 out]
            n125 = property on="Ch No" class="DigNum (strict)"("Disabled"=w288) -> ()  [unwired: 2 in, 2 out]
            n126 = property on="high limit (10V)" class="DigNum (strict)"("Disabled"=w287) -> ()  [unwired: 2 in, 2 out]
            n127 = property on="low limit (-10V)" class="DigNum (strict)"("Disabled"=w286) -> ()  [unwired: 2 in, 2 out]
            n128 = property on="Off ch no" class="DigNum (strict)"("Disabled"=w285) -> ()  [unwired: 2 in, 2 out]
          }
          frame #6 {
            n129 = Unbundle By Name(w360) -> ("Ref Instrument type"=w359:T3)
            n130 = Index Array(array=w357, index=w359) -> (element=w358:string)
          }
          frame #7 {
            n131 = Unbundle By Name(w364) -> ("Ref Instrument type"=w365:T3)
            n132 = case shown="\"Pitot-static tube\"" w365 {
              tunnel: [u8 0 u8 0 u8 0 u8 0 u8 0 u8 0 u8 0 u8 0 u8 2 u8 2 u8 2] -> w366
              tunnel: [u8 0 u8 0 u8 2 u8 0 u8 0 u8 0 u8 0 u8 0 u8 2 u8 2 u8 2] -> w370
              tunnel: [u8 0 u8 0 u8 0 u8 0 u8 0 u8 0 u8 0 u8 0 u8 2 u8 2 u8 2] -> w369
              tunnel: [u8 0 u8 0 u8 0 u8 0 u8 0 u8 0 u8 0 u8 0 u8 2 u8 2 u8 2] -> w368
              tunnel: [u8 0 u8 0 u8 0 u8 0 u8 0 u8 0 u8 0 u8 0 u8 2 u8 2 u8 2] -> w367
              tunnel: [enum16{"No 2nd ref inst", "Add 2nd ref inst"}."Add 2nd ref inst" enum16{"No 2nd ref inst", "Add 2nd ref inst"}."Add 2nd ref inst" enum16{"No 2nd ref inst", "Add 2nd ref inst"}."Add 2nd ref inst" enum16{"No 2nd ref inst", "Add 2nd ref inst"}."Add 2nd ref inst" enum16{"No 2nd ref inst", "Add 2nd ref inst"}."Add 2nd ref inst" enum16{"No 2nd ref inst", "Add 2nd ref inst"}."Add 2nd ref inst" enum16{"No 2nd ref inst", "Add 2nd ref inst"}."Add 2nd ref inst" enum16{"No 2nd ref inst", "Add 2nd ref inst"}."Add 2nd ref inst" enum16{"No 2nd ref inst", "Add 2nd ref inst"}."No 2nd ref inst" enum16{"No 2nd ref inst", "Add 2nd ref inst"}."No 2nd ref inst" enum16{"No 2nd ref inst", "Add 2nd ref inst"}."No 2nd ref inst"] -> w361
              frame "Propellor anemometer" {
              }
              frame "Pressure Transducer" {
              }
              frame "Raw voltage" {
              }
              frame "Pitot-static tube" {
              }
              frame "Preston tube" {
              }
              frame "Generic Linear" {
              }
              frame "Generic Polynomial" {
              }
              frame "Thermocouple" {
              }
              frame "LDA" {
              }
              frame "Enter Value" {
              }
              frame "ADAM Channel" {
              }
            }
            n133 = case shown="\"Cross wire angle\"" w363 {
              tunnel: [w371 enum16{"No 2nd ref inst", "Add 2nd ref inst"}."No 2nd ref inst"] -> w362
              tunnel: w361 -> [w371 _]
              frame "Cross wire angle" {
              }
              frame "Generic Linear", Default {
              }
            }
            n134 = property on="Calib filename" class="Path"("Disabled"=w370) -> ()  [unwired: 2 in, 2 out]
            n135 = property on="low limit (-10V)" class="DigNum (strict)"("Disabled"=w369) -> ()  [unwired: 2 in, 2 out]
            n136 = property on="high limit (10V)" class="DigNum (strict)"("Disabled"=w368) -> ()  [unwired: 2 in, 2 out]
            n137 = property on="Ch No" class="DigNum (strict)"("Disabled"=w367) -> ()  [unwired: 2 in, 2 out]
            n138 = property on="Off ch no" class="DigNum (strict)"("Disabled"=w366) -> ()  [unwired: 2 in, 2 out]
          }
          frame #8 {
            n139 = for {
              tunnel: w441 -> [w449] mode=indexing
              tunnel: [w447] -> w440 mode=indexing
              tunnel: w439 -> [w443] mode=indexing
              n140 = Unbundle By Name(w443) -> ("high limit (10V)"=w446:sgl, "low limit (-10V)"=w445:sgl, "Ch No"=w444:i16, "DAQmx Channel"=w442:tag)
              n141 = Bundle By Name(cluster="Type", "high limit (10V)"=w446, "low limit (-10V)"=w445, "Ch No"=w444, "Var name"=w449, "DAQmx Chan"=w442) -> (w447:T1)
            }
          }
          frame #9 {
            n142 = local read "Type"() -> (w455:T1)
            n143 = case shown="1.." w459 {
              tunnel: [w463 w487] -> w450
              tunnel: w458 -> [w466 w481]
              tunnel: w451 -> [_ w484]
              tunnel: w457 -> [_ w483]
              tunnel: [w465 w486] -> w456
              tunnel: w455 -> [w464 w485]
              tunnel: w452 -> [w460 _]
              tunnel: w454 -> [w462 _]
              tunnel: w453 -> [w461 _]
              frame ..0 {
                n144 = case shown="\"Add 2nd ref inst\"" w462 {
                  tunnel: [w468 w479] -> w463
                  tunnel: w461 -> [_ w469]
                  tunnel: w460 -> [_ w478]
                  tunnel: w464 -> [_ w477]
                  tunnel: [path "" w476] -> w465
                  tunnel: w466 -> [w468 w471]
                  frame "No 2nd ref inst" {
                  }
                  frame "Add 2nd ref inst" {
                    n145 = Unbundle By Name(w478) -> ("high limit (10V)"=w473:sgl, "low limit (-10V)"=w474:sgl, "Ch No"=w475:i16, "Calib filename"=w476:path, "DAQmx Channel"=w470:tag)
                    n146 = Bundle By Name(cluster=w477, "high limit (10V)"=w473, "low limit (-10V)"=w474, "Ch No"=w475, "DAQmx Chan"=w470, "Var name"=w469) -> (w472:T1)
                    n147 = Build Array (concatenate)(w472, w471) -> (w479:T1[])
                  }
                }
              }
              frame 1.. {
                n148 = Unbundle By Name(w484) -> ("high limit (10V)"=w490:sgl, "low limit (-10V)"=w489:sgl, "Ch No"=w488:i16, "Calib filename"=w486:path, "DAQmx Channel"=w480:tag)
                n149 = Bundle By Name(cluster=w485, "high limit (10V)"=w490, "low limit (-10V)"=w489, "Ch No"=w488, "Var name"=w483, "DAQmx Chan"=w480) -> (w482:T1)
                n150 = local write "Type"(w482) -> ()
                n151 = Build Array (concatenate)(w482, w481) -> (w487:T1[])
              }
            }
          }
          frame #10 {
            n152 = case shown="True" "Edit temp and Press" {
              frame False {
              }
              frame True {
                n153 = stacked-sequence {
                  frame #0 {
                    w492 = TRUE  # Wait until done
                    n154 = call "Run_Enter_Temp.vi"("Wait until done"=w492) -> ()  [unwired: 1 out]
                  }
                  frame #1 {
                    n155 = call "Get_Temp_and_Press.vi"("Averaging time (mins)"=0.5) -> ("Abs Press (mbar)"=w494:dbl, "Temperature"=w493:dbl)  [unwired: 3 out]
                    n156 = local write "Abs Press (mbar)"(w494) -> ()
                    n157 = local write "Temp (deg C)"(w493) -> ()
                  }
                }
              }
            }
          }
          frame #11 {
            # "#optimation Should probably also check for duplicate DAQmx Channels"
            n158 = case shown="True" "OK" {
              tunnel: w498 -> [_ w502]
              tunnel: [TRUE w501] -> w496
              frame False {
              }
              frame True {
                n159 = stacked-sequence {
                  seq-local: [w503 _] -> [_ w521]
                  tunnel: w502 -> [w505 w523]
                  tunnel: [_ w519] -> w501
                  frame #0 {
                    n160 = for {
                      shift-right: [w512] -> _
                      shift-left: i16[] [] -> [w511]
                      tunnel: w505 -> [w508] mode=indexing
                      tunnel: [w507] -> w504 mode=indexing
                      n161 = Unbundle By Name(w508) -> ("Ch No"=w509:i16)
                      n162 = Search 1D Array(1D array=w511, element=w509) -> (index of element=w510:i32)  [unwired: 1 out]
                      n163 = Build Array (concatenate)(w511, w509) -> (w512:i16[])
                      n164 = case shown="0, Default" w510 {
                        tunnel: w509 -> [w517 _]
                        tunnel: [w513 FALSE ("true")] -> w507
                        frame 0, Default {
                          n165 = Format Into String(format string="The Ch No %d appears more than once", w517) -> (resulting string=w515:string)  [unwired: 2 in, 1 out]
                          n166 = One Button Dialog(message=w515, button name ("OK")="Ok") -> (true=w513:bool)
                        }
                        frame -1 {
                        }
                      }
                    }
                    n167 = Or Array Elements(Boolean array=w504) -> (logical OR=w503:bool)
                  }
                  frame #1 {
                    n168 = for {
                      tunnel: w523 -> [w529] mode=indexing
                      tunnel: [w528] -> w522 mode=indexing
                      n169 = Unbundle By Name(w529) -> ("high limit (10V)"=w527:sgl, "low limit (-10V)"=w526:sgl, "Ch No"=w524:i16)
                      n170 = Greater Or Equal?(x=w527, y=w526) -> (x >= y?=w525:bool)
                      n171 = case shown="False" w525 {
                        tunnel: [TRUE ("true") FALSE ("true")] -> w528
                        tunnel: w524 -> [w531 _]
                        frame False {
                          n172 = Number To Decimal String(number=w531) -> (decimal integer string=w532:string)  [unwired: 1 out]
                          n173 = Concatenate Strings("Error in input limits for Channel No ", w532) -> (w533:string)
                          n174 = One Button Dialog(message=w533) -> ()  [unwired: 2 out]
                        }
                        frame True {
                        }
                      }
                    }
                    n175 = Or Array Elements(Boolean array=w522) -> (logical OR=w520:bool)
                    n176 = Or(x=w520, y=w521) -> (x .or. y?=w519:bool)
                  }
                }
              }
            }
          }
          frame #12 {
            n177 = Unbundle By Name(w539) -> ("Ref Instrument type"=w538:T3)
            n178 = Equal?(x=Ref_Inst_type."Preston tube" ("Ref Instrument type"), y=w538) -> (x = y?=w536:bool)
            n179 = property on="Preston tube diammeter in mm" class="DigNum (strict)"("Visible"=w536) -> ()  [unwired: 2 in, 2 out]
          }
        }
      }
      "Instrument type" <- w71
      "Calib filename" <- w73
      "Ch & Spans" <- w64
      n180 = global write "Calib_global.vi" "Angle/vel calib file"(w68) -> ()
      n181 = global write "Calib_global.vi" "existing angle calib"(w67) -> ()
    }
    frame #4 {
      n182 = global read "Calib_global.vi" "Pre Setup String"() -> (w541:string)
      n183 = case shown="\"Setup Front Panel\"" w546 {
        tunnel: [w548 w558] -> w545
        tunnel: "Sampling speeds" -> [w548 w560]
        tunnel: [w547 w554] -> w543
        tunnel: "Fixed n" -> [w547 _]
        tunnel: w541 -> [_ w553]
        tunnel: w540 -> [_ _]
        frame "Show Setup", Default {
        }
        frame "Setup Front Panel" {
          n184 = call "Get_value_from_string.vi"("Input string"=w553, "Variable name"="Requested sampling rate") -> ("Status"=w551:enum16{"Char in string", "Char not in string"}, "Value"=w549:dbl)  [unwired: 1 in]
          n185 = case shown="\"Char not in string\"" w551 {
            tunnel: [w562 sgl 100.0 ("Sampling Rate /ch (Hz)")] -> w550
            tunnel: w549 -> [w562 _]
            frame "Char in string" {
            }
            frame "Char not in string" {
            }
          }
          n186 = call "Get_value_from_string.vi"("Input string"=w553, "Variable name"="No of samples") -> ("Value"=w559:dbl)  [unwired: 1 in, 1 out]
          n187 = call "Get_Characters_from_string.vi"("Input string"=w553, "Variable name"="Fixed Coefficient n") -> ("Value"=w556:string)  [unwired: 1 in, 1 out]
          n188 = Equal?(x="TRUE", y=w556) -> (x = y?=w554:bool)
          n189 = Bundle By Name(cluster=w560, "Samples /ch"=w559, "Sampling Rate /ch (Hz)"=w550) -> (w558:T6)
        }
      }
      "Sampling speeds Output" <- w545
      "Fixed n out" <- w543
    }
    frame #5 {
      n190 = property on="Calib filename" class="Path"() -> ("Disabled"=w568:u8)  [unwired: 2 in, 2 out]
      n191 = Equal To 0?(x=w568) -> (x = 0?=w567:bool)
      n192 = local read "Reference instrument"() -> (w566:T8)
      n193 = case shown="True" w567 {
        tunnel: w566 -> [w571 w577]
        tunnel: [w570 w576] -> w565
        tunnel: w564 -> [_ w572]
        frame False {
          n194 = Bundle By Name(cluster=w571, "Calib filename"=path "") -> (w570:T8)
        }
        frame True {
          w573 = FALSE  # Use Latest Calib
          n195 = Unbundle By Name(w577) -> ("Calib filename"=w579:path, "Ref Instrument type"=w575:T3)
          n196 = case shown="\"Generic Polynomial\"" w575 {
            tunnel: [Inst_type."Propeller anemometer" ("Inst type") Inst_type."Pressure Transducer" ("Inst type") Inst_type."Pressure Transducer" ("Inst type") Inst_type."Pitot-static tube" ("Inst type") Inst_type."Preston tube" ("Inst type") Inst_type."Generic Linear" ("Inst type") Inst_type."Generic Polynomial" ("Inst type") Inst_type."Thermocouple" ("Inst type") Inst_type."Raw voltage" ("Inst type") Inst_type."Raw voltage" ("Inst type") Inst_type."Raw voltage" ("Inst type")] -> w574
            frame "Propellor anemometer" {
            }
            frame "Pressure Transducer" {
            }
            frame "Raw voltage" {
            }
            frame "Pitot-static tube" {
            }
            frame "Preston tube" {
            }
            frame "Generic Linear" {
            }
            frame "Generic Polynomial" {
            }
            frame "Thermocouple" {
            }
            frame "LDA" {
            }
            frame "Enter Value" {
            }
            frame "ADAM Channel" {
            }
          }
          n197 = case shown="\"Take a New Calibration Point\", Default" w572 {
            tunnel: w579 -> [w580 w584]
            tunnel: [w580 w583] -> w578
            tunnel: w574 -> [_ w582]
            tunnel: w573 -> [_ w581]
            frame "Refit Curve" {
            }
            frame "Take a New Calibration Point", Default {
              n198 = call "Find_calibration_file.vi"("Inst type"=w582, "Use Latest Calib"=w581, "filename"=w584) -> ("filename out"=w583:path)  [unwired: 1 in]
            }
          }
          n199 = Bundle By Name(cluster=w577, "Calib filename"=w578) -> (w576:T8)
        }
      }
      n200 = local write "Reference instrument"(w565) -> ()
    }
    frame #6 {
      n201 = property on="Ref vel for angle calib" class="Clust (strict)"() -> ("Disabled"=w596:u8)  [unwired: 2 in, 2 out]
      n202 = local read "Ref vel for angle calib"() -> (w598:T8)
      n203 = case shown="0" w596 {
        tunnel: w598 -> [w603 w619]
        tunnel: [w602 w618] -> w597
        frame 0 {
          w599 = FALSE  # Use Latest Calib
          n204 = Unbundle By Name(w603) -> ("Calib filename"=w605:path, "Ref Instrument type"=w601:T3)
          n205 = case shown="\"LDA\"" w601 {
            tunnel: [Inst_type."Propeller anemometer" ("Inst type") Inst_type."Pressure Transducer" ("Inst type") Inst_type."Pressure Transducer" ("Inst type") Inst_type."Pitot-static tube" ("Inst type") Inst_type."Preston tube" ("Inst type") Inst_type."Generic Linear" ("Inst type") Inst_type."Generic Polynomial" ("Inst type") Inst_type."Thermocouple" ("Inst type") Inst_type."Raw voltage" ("Inst type") Inst_type."Raw voltage" ("Inst type") Inst_type."Raw voltage" ("Inst type")] -> w600
            frame "Propellor anemometer" {
            }
            frame "Pressure Transducer" {
            }
            frame "Raw voltage" {
            }
            frame "Pitot-static tube" {
            }
            frame "Preston tube" {
            }
            frame "Generic Linear" {
            }
            frame "Generic Polynomial" {
            }
            frame "Thermocouple" {
            }
            frame "LDA" {
            }
            frame "Enter Value" {
            }
            frame "ADAM Channel" {
            }
          }
          n206 = call "Find_calibration_file.vi"("Inst type"=w600, "Use Latest Calib"=w599, "filename"=w605) -> ("filename out"=w604:path)  [unwired: 1 in]
          n207 = Bundle By Name(cluster=w603, "Calib filename"=w604) -> (w602:T8)
        }
        frame 1, Default {
          n208 = Bundle By Name(cluster=w619, "Calib filename"=path "") -> (w618:T8)
        }
      }
      n209 = local write "Ref vel for angle calib"(w597) -> ()
    }
    frame #7 {
      w626 = Ref_Inst_type."ADAM Channel" ("Ref Instrument type")
      n210 = global write "Calib_global.vi" "Ref Instrument type"(w623) -> ()
      n211 = local read "Ref vel for angle calib"() -> (w628:T8)
      n212 = property on="Ref vel for angle calib" class="Clust (strict)"() -> ("Disabled"=w621:u8)  [unwired: 2 in, 2 out]
      n213 = Unbundle By Name(w628) -> ("Ref Instrument type"=w627:T3)
      n214 = Equal To 0?(x=w621) -> (x = 0?=w620:bool)
      n215 = Equal?(x=w623, y=w626) -> (x = y?=w625:bool)
      n216 = local read "2nd ref instrument"() -> (w629:T7)
      n217 = Bundle By Name(cluster=w629, "2nd Ref type"=w627, "2nd inst present"=w620) -> (→"2nd ref instrument":T7)
      n218 = case shown="True" w620 {
        tunnel: w627 -> [_ w635]
        tunnel: w626 -> [_ w634]
        tunnel: w625 -> [w630 w632]
        tunnel: [w630 w631] -> w624
        frame False {
        }
        frame True {
          n219 = Equal?(x=w635, y=w634) -> (x = y?=w633:bool)
          n220 = Or(x=w633, y=w632) -> (x .or. y?=w631:bool)
        }
      }
    }
    frame #8 {
      n221 = Equal?(x=Calib_mode."Show Setup" ("Mode"), y=w643) -> (x = y?=w642:bool)
      n222 = And(x=w642, y=w641) -> (x .and. y?=w640:bool)
      n223 = global read "Calib_global.vi" "Pre Setup String"() -> (w639:string)
      n224 = case shown="True" w640 {
        tunnel: [w646 w652] -> w644
        tunnel: w639 -> [w648 w651]
        tunnel: "ADAM Channel name" -> [w647 w650]
        tunnel: [w645 w649] -> w637
        frame False {
          n225 = call "Get_Characters_from_string.vi"("Input string"=w648, "Variable name"=w647) -> ("Value"=w645:string)  [unwired: 1 in, 1 out]
          n226 = call "Characters_to_string.vi"("Characters to write"=w645, "Label for characters"=w647) -> ("Output string"=w646:string)
        }
        frame True {
          n227 = stacked-sequence {
            seq-local: [_ w656 _ _ _ _] -> [_ _ _ w666 _ _]
            seq-local: [_ _ _ w660 _ _] -> [_ _ _ _ _ _]
            seq-local: [_ _ w658 _ _ _] -> [_ _ _ _ _ w676]
            tunnel: [_ _ _ _ _ w675] -> w652
            tunnel: w651 -> [_ _ _ _ _ w671]
            tunnel: w650 -> [_ _ _ _ _ w670]
            tunnel: [_ _ _ _ _ w669] -> w649
            frame #0 {
              n228 = property on="Message" class="Str"("Visible"=TRUE) -> ()  [unwired: 2 in, 2 out]
              "Message" <- "Message\n\nCurrently trying to connect to the server.\n\nPlease Wait"
            }
            frame #1 {
              n229 = Get Date/Time In Seconds() -> (seconds since 1Jan1904=w655:timestamp)
              n230 = To Double Precision Float(number=w655) -> (double precision float=w656:dbl)
            }
            frame #2 {
              n231 = call "Get_ADAM_Ch_names_client.vi"("Channel names set"=Channel_names."Active Only") -> ("Ch names"=w658:string[])
            }
            frame #3 {
              n232 = Get Date/Time In Seconds() -> (seconds since 1Jan1904=w659:timestamp)
              n233 = To Double Precision Float(number=w659) -> (double precision float=w665:dbl)
              n234 = Subtract(x=w665, y=w666) -> (x-y=w664:dbl)
              n235 = Number To Decimal String(number=w664) -> (decimal integer string=w662:string)  [unwired: 1 out]
              n236 = Concatenate Strings("Server took ", w662, " Seconds to respond") -> (w660:string)
            }
            frame #4 {
              n237 = property on="Message" class="Str"("Visible"=FALSE) -> ()  [unwired: 2 in, 2 out]
            }
            frame #5 {
              n238 = call "Get_Characters_from_string.vi"("Input string"=w671, "Variable name"=w670) -> ("Status"=w674:enum16{"Char in string", "Char not in string"}, "Value"=w673:string)  [unwired: 1 in]
              n239 = case shown="\"Char in string\"" w674 {
                tunnel: w673 -> [w677 _]
                tunnel: [w677 "" ("Value")] -> w672
                frame "Char in string" {
                }
                frame "Char not in string" {
                }
              }
              n240 = call "Select_Single_ADAM_Ch.vi"("Desired Ch name (in)"=w672, "Available Ch names"=w676, "Message"="Please Choose Reference Instrument") -> ("Ch Name"=w669:string)  [unwired: 3 out]
              n241 = call "Characters_to_string.vi"("Characters to write"=w669, "Label for characters"=w670) -> ("Output string"=w675:string)
            }
          }
        }
      }
      n242 = global write "Calib_global.vi" "ADAM Channel Name"(w637) -> ()
    }
    frame #9 {
      n243 = local read "2nd ref instrument"() -> (w685:T7)
      n244 = Equal?(x=Calib_mode."Show Setup" ("Mode"), y=w692) -> (x = y?=w691:bool)
      n245 = Unbundle By Name(w685) -> ("2nd Ref type"=w683:T3, "2nd inst present"=w681:bool)
      n246 = global read "Calib_global.vi" "Pre Setup String"() -> (w689:string)
      n247 = Equal?(x=Ref_Inst_type."ADAM Channel" ("2nd Ref type"), y=w683) -> (x = y?=w682:bool)
      n248 = And(x=w682, y=w681) -> (x .and. y?=w680:bool)
      n249 = And(x=w691, y=w680) -> (x .and. y?=w690:bool)
      n250 = case shown="True" w690 {
        tunnel: [w694 w700] -> w679
        tunnel: w689 -> [w696 w699]
        tunnel: "ADAM Channel name for 2nd Ref Instr" -> [w695 w698]
        tunnel: [w693 w697] -> w687
        frame False {
          n251 = call "Get_Characters_from_string.vi"("Input string"=w696, "Variable name"=w695) -> ("Value"=w693:string)  [unwired: 1 in, 1 out]
          n252 = call "Characters_to_string.vi"("Characters to write"=w693, "Label for characters"=w695) -> ("Output string"=w694:string)
        }
        frame True {
          n253 = stacked-sequence {
            seq-local: [_ w704 _ _ _ _] -> [_ _ _ w714 _ _]
            seq-local: [_ _ _ w708 _ _] -> [_ _ _ _ _ _]
            seq-local: [_ _ w706 _ _ _] -> [_ _ _ _ _ w724]
            tunnel: [_ _ _ _ _ w723] -> w700
            tunnel: w699 -> [_ _ _ _ _ w719]
            tunnel: w698 -> [_ _ _ _ _ w718]
            tunnel: [_ _ _ _ _ w717] -> w697
            frame #0 {
              n254 = local write "Message"("Message\n\nCurrently trying to connect to the server.\n\nPlease Wait") -> ()
              n255 = property on="Message" class="Str"("Visible"=TRUE) -> ()  [unwired: 2 in, 2 out]
            }
            frame #1 {
              n256 = Get Date/Time In Seconds() -> (seconds since 1Jan1904=w703:timestamp)
              n257 = To Double Precision Float(number=w703) -> (double precision float=w704:dbl)
            }
            frame #2 {
              n258 = call "Get_ADAM_Ch_names_client.vi"("Channel names set"=Channel_names."Active Only") -> ("Ch names"=w706:string[])
            }
            frame #3 {
              n259 = Get Date/Time In Seconds() -> (seconds since 1Jan1904=w707:timestamp)
              n260 = To Double Precision Float(number=w707) -> (double precision float=w713:dbl)
              n261 = Subtract(x=w713, y=w714) -> (x-y=w712:dbl)
              n262 = Number To Decimal String(number=w712) -> (decimal integer string=w710:string)  [unwired: 1 out]
              n263 = Concatenate Strings("Server took ", w710, " Seconds to respond") -> (w708:string)
            }
            frame #4 {
              n264 = property on="Message" class="Str"("Visible"=FALSE) -> ()  [unwired: 2 in, 2 out]
            }
            frame #5 {
              n265 = call "Get_Characters_from_string.vi"("Input string"=w719, "Variable name"=w718) -> ("Status"=w722:enum16{"Char in string", "Char not in string"}, "Value"=w721:string)  [unwired: 1 in]
              n266 = case shown="\"Char in string\"" w722 {
                tunnel: w721 -> [w725 _]
                tunnel: [w725 "" ("Value")] -> w720
                frame "Char in string" {
                }
                frame "Char not in string" {
                }
              }
              n267 = call "Select_Single_ADAM_Ch.vi"("Desired Ch name (in)"=w720, "Available Ch names"=w724, "Message"="Please Choose 2nd Ref Channel") -> ("Ch Name"=w717:string)  [unwired: 3 out]
              n268 = call "Characters_to_string.vi"("Characters to write"=w717, "Label for characters"=w718) -> ("Output string"=w723:string)
            }
          }
        }
      }
      n269 = global write "Calib_global.vi" "ADAM Channel Name Vel Ref"(w687) -> ()
    }
    frame #10 {
      n270 = local read "Reference instrument"() -> (w731:T8)
      n271 = local read "2nd ref instrument"() -> (w732:T7)
      n272 = local read "Sampling speeds Output"() -> (w728:T6)
      n273 = local read "Abs Press (mbar)"() -> (w729:dbl)
      n274 = local read "Temp (deg C)"() -> (w727:dbl)
      n275 = global write "Calib_global.vi" "2nd ref instrument"(w732) -> ()
      n276 = Unbundle By Name(w728) -> ("Sampling Rate /ch (Hz)"=w734:sgl, "Samples /ch"=w735:i32)
      n277 = global write "Calib_global.vi" "Abs Press (mbar)"(w729) -> ()
      n278 = global write "Calib_global.vi" "Temp (deg C)"(w727) -> ()
      n279 = call "Calib_General_Setup.vi"("Reference instrument"=w731, "Requested No of samples"=w735, "Sampling rate (Hz)"=w734, "2nd ref instrument"=w732, "Temp"=w727, "Abs Press (mbar)"=w729) -> ("Output string"=w733:string, "LDA Data"=w730:bool)  [unwired: 8 out]
    }
    frame #11 {
      n280 = local read "Ref vel for angle calib"() -> (w744:T8)
      n281 = local read "Reference instrument"() -> (w743:T8)
      n282 = local read "Instrument type"() -> (w742:T9)
      n283 = global write "Calib_global.vi" "Instrument type"(w742) -> ()
      n284 = case shown="\"Propeller anemometer\", Default" w742 {
        tunnel: [w747 w748 w750] -> w741
        tunnel: w744 -> [w746 w749 _]
        tunnel: [w746 w749 w750] -> w737
        tunnel: w743 -> [w747 w748 w750]
        frame "Propeller anemometer", Default {
        }
        frame "Cross wire angle" {
        }
        frame "Cross wire velocity" {
        }
      }
      n285 = call "Reference_Inst_Info_2_string.vi"("Reference instrument"=w741, "Reference Name"="Reference instrument") -> ("Setup String"=w739:string)
      n286 = call "Reference_Inst_Info_2_string.vi"("Reference instrument"=w737, "Reference Name"="Ref vel for angle calib") -> ("Setup String"=w736:string)
      n287 = Concatenate Strings(w739, w736) -> (w745:string)
    }
    frame #12 {
      n288 = local read "Instrument type"() -> (w751:T9)
      n289 = case shown="\"Pulsed Wire\"" w751 {
        tunnel: ["" w760] -> w752
        tunnel: w753 -> [_ w759]
        frame "Propeller anemometer", Default {
        }
        frame "Pulsed Wire" {
          w755 = FALSE  # Check Calib file?
          n290 = case shown="\"Refit Curve\", Default" w759 {
            tunnel: [w762 w764] -> w758
            tunnel: [w761 w763] -> w757
            frame "Refit Curve", Default {
              w762 = FALSE  # Show Panel?
              w761 = T12 TRUE  # OK
            }
            frame "Show Setup" {
              w764 = TRUE  # Show Panel?
              w763 = T12 FALSE  # OK
            }
          }
          n291 = global read "Calib_global.vi" "Pre Setup String"() -> (w756:string)
          n292 = call "PWA_Setup_Panel.vi"("Show Panel?"=w758, "Check Calib file?"=w755, "OK"=w757, "Incoming Setup String"=w756) -> ("Outgoing Setup String"=w760:string)  [unwired: 3 out]
        }
      }
    }
    frame #13 {
      n293 = local read "instrument to calibrate"() -> (w770:T11)
      n294 = global read "Meas_global.vi" "Acquisition vi to Run"() -> (w767:string)
      n295 = for {
        tunnel: w770 -> [w805] mode=indexing
        shift-right: [w790] -> w773
        shift-left: "" -> [w794]
        i -> [w804]
        n296 = Increment(x=w804) -> (x+1=w789:i32)
        n297 = Unbundle By Name(w805) -> ("high limit (10V)"=w801:sgl, "low limit (-10V)"=w796:sgl, "Ch No"=w795:i16, "DAQmx Channel"=w783:tag)
        n298 = Format Into String(format string="Inst_to_calibrate_element_%d ", w789) -> (resulting string=w784:string)  [unwired: 2 in, 1 out]
        n299 = Concatenate Strings(w784, "Low limit") -> (w800:string)
        n300 = Concatenate Strings(w784, "Ch No") -> (w799:string)
        n301 = Concatenate Strings(w784, "DAQ Ch") -> (w785:string)
        n302 = Concatenate Strings(w784, "High limit") -> (w802:string)
        n303 = call "Characters_to_string.vi"("Characters to write"=w783, "Label for characters"=w785) -> ("Output string"=w787:string)
        n304 = call "Value_to_string.vi"("Value"=w796, "Label for value"=w800) -> ("Output string"=w792:string)  [unwired: 1 in]
        n305 = call "Value_to_string.vi"("Value"=w795, "Label for value"=w799) -> ("Output string"=w791:string)  [unwired: 1 in]
        n306 = call "Value_to_string.vi"("Value"=w801, "Label for value"=w802) -> ("Output string"=w793:string)  [unwired: 1 in]
        n307 = Concatenate Strings(w794, w793, w792, w791, w787) -> (w790:string)
      }
      n308 = Array Size(array=w770) -> (size(s)=w769:i32)
      n309 = Equal To 0?(x=w769) -> (x = 0?=w768:bool)
      n310 = Equal?(x=w767, y="NI-DAQmx.vi") -> (x = y?=w765:bool)
      n311 = case shown="False" w768 {
        tunnel: [w776 "-10" ("Ch No")] -> w771
        tunnel: w770 -> [w779 _]
        tunnel: w765 -> [w774 _]
        frame False {
          w781 = 0  # index
          n312 = Index Array(array=w779, index=w781) -> (element=w780:T18)
          n313 = Unbundle By Name(w780) -> ("Ch No"=w778:i16, "DAQmx Channel"=w775:tag)
          n314 = Number To Decimal String(number=w778) -> (decimal integer string=w777:string)  [unwired: 1 in]
          n315 = Select(t=w775, s=w774, f=w777) -> (s? t:f=w776:string)
        }
        frame True {
        }
      }
      n316 = global write "Calib_global.vi" "Calib Ch No"(w771) -> ()
    }
    frame #14 {
      n317 = local read "Preston tube diammeter in mm"() -> (w809:dbl)
      n318 = local read "Instrument type"() -> (w820:T9)
      n319 = property on="Instrument type" class="Enum (strict)"() -> ("Strings []"=w821:string[])  [unwired: 2 in, 2 out]
      n320 = local read "angle calib"() -> (w814:T10)
      n321 = property on="angle calib" class="Enum (strict)"() -> ("Strings []"=w815:string[])  [unwired: 2 in, 2 out]
      n322 = Index Array(array=w821, index=w820) -> (element=w819:string)
      n323 = Index Array(array=w815, index=w814) -> (element=w813:string)
      n324 = call "Characters_to_string.vi"("Characters to write"=w819, "Label for characters"="Instrument_type_to Calibrate") -> ("Output string"=w817:string)
      n325 = call "Value_to_string.vi"("Value"=w809, "Label for value"="Preston tube diameter in mm" ("Variable name")) -> ("Output string"=w808:string)  [unwired: 1 in]
      n326 = call "Characters_to_string.vi"("Characters to write"=w813, "Label for characters"="Angle calib") -> ("Output string"=w812:string)
      n327 = local read "Fixed n out"() -> (w825:bool)
      n328 = Concatenate Strings(w808, w817, w812) -> (w832:string)
      n329 = Select(t="TRUE", s=w825, f="FALSE") -> (s? t:f=w826:string)
      n330 = global read "Calib_global.vi" "New Setup String"() -> (w824:string)
      n331 = call "Characters_to_string.vi"("Characters to write"=w826, "Label for characters"="Fixed Coefficient n") -> ("Output string"=w822:string)
      n332 = Concatenate Strings(w824, w822, w832, w831, w806, w830, w807, w823, w811) -> (w833:string)
      n333 = global write "Calib_global.vi" "New Setup String"(w833) -> ()
    }
    frame #15 {
      n334 = Equal?(x=Calib_mode."Show Setup" ("Mode"), y=w839) -> (x = y?=w838:bool)
      n335 = And(x=w837, y=w838) -> (x .and. y?=w836:bool)
      n336 = case shown="True" w836 {
        tunnel: [FALSE ("Synchronise with LDA") FALSE ("Synchronise with LDA")] -> w834
        frame False {
        }
        frame True {
          n337 = global read "LDA_meas_global_1.vi" "BSA Type"() -> (w843:T19)
          n338 = case shown="\"BSA F60\"" w843 {
            tunnel: TRUE -> [_ w853]
            frame "57N11" {
              n339 = stacked-sequence {
                frame #0 {
                  n340 = Bundle By Name(cluster=T16 {"dimensions"=enum."2D", "Analogue Freq Multiplier"=0.1} ("LDA set up"), "dimensions"=enum16{"1D", "2D"}."1D", "Analogue Freq Multiplier"=2.0) -> (w846:T16)
                  n341 = global write "Meas_global.vi" "LDA set up"(w846) -> ()
                }
                frame #1 {
                  w848 = "1"  # BSA Number
                  n342 = call "Control_BSA_setup.vi"("setup"=Setup."Show Setup", "BSA number"=w848) -> ()  [unwired: 14 out]
                }
                frame #2 {
                  n343 = global read "LDA_meas_global_2.vi" "BSA2 info"() -> (w850:T20)
                  n344 = Unbundle By Name(w850) -> ("GPIB Address"=w851:string)
                  n345 = call "Set_BSA_Coincidence.vi"("GPIB address"=w851, "Set Coincidence"=enum16{"Slave", "Master", "Private"}."Slave") -> ()  [unwired: 1 in, 5 out]
                }
              }
            }
            frame "BSA F60" {
              n346 = disable-structure shown="TARGET_TYPE==Windows" {
                disable-tunnel: w853 -> [_ w854]
                frame condition #0 {
                }
                frame condition #1 (active) {
                  n347 = call "Edit_BSA_IP.vi"("Show Panel"=w854) -> ()  [unwired: 3 out]
                }
              }
            }
          }
        }
      }
      n348 = global write "Meas_global.vi" "Synchronise with LDA"(w834) -> ()
    }
    frame #16 {
      w863 = TRUE  # Lock File
      w872 = FALSE  # advisory dialog? (display:T)
      w873 = FALSE  # append to file? (new file:F)
      n349 = local read "Ch & Spans"() -> (w855:T1[])
      n350 = local read "Instrument type"() -> (w861:T9)
      n351 = local read "Calib filename"() -> (w874:path)
      n352 = global read "Meas_global.vi" "LDA data"() -> (w866:enum16{"No LDA data", "Take LDA data"})
      n353 = global write "Calib_global.vi" "Ref Calib file"(w874) -> ()
      n354 = case shown="\"Take LDA data\"" w866 {
        tunnel: ["" w883] -> w864
        frame "No LDA data" {
        }
        frame "Take LDA data" {
          w882 = ""  # Used to be LDA-header.vi
          n355 = call "LDA_U16_data_header.vi"() -> ("Output string"=w884:string)  [unwired: 1 out]
          n356 = Concatenate Strings(w882, w884) -> (w883:string)
        }
      }
      n357 = case shown="\"Pulsed Wire\"" w861 {
        tunnel: ["" w876] -> w860
        frame "Propeller anemometer", Default {
        }
        frame "Pulsed Wire" {
          n358 = property on="PWA Data" class="Enum (strict)"() -> ("Strings []"=w879:string[])  [unwired: 2 in, 2 out]
          n359 = Index Array(array=w879, index=PWA_Data."One Ch PWA" ("PWA Data")) -> (element=w877:string)
          n360 = call "Characters_to_string.vi"("Characters to write"=w877, "Label for characters"="Pulsed_Wire_Data" ("Variable name")) -> ("Output string"=w876:string)
        }
      }
      n361 = call "Calib_Ch_setup.vi"("Preston tube diammeter in mm"="Preston tube diammeter in mm", "Ch & Spans"=w855, "Calib filename"=w874) -> ("Output string"=w867:string)
      n362 = global write "Calib_global.vi" "Ch & Spans"(w855) -> ()
      n363 = call "Date_and_Time_to_string.vi"() -> ("Date and time (spreadsheet)"=w865:string)
      n364 = Concatenate Strings(w865, w860, w864, w868, w867, w859) -> (w869:string)
      n365 = call "Setup_Filepath.vi"("Setup File Type"=Setup_Filetype."Measurement Setups", "Filename in"="Calib_Setup.xls") -> ("Filename Out"=w856:path)  [unwired: 1 out]
      n366 = call "Add_label_to_string.vi"("String to write"=w869, "File Label"="Raw data header") -> ("Output string"=w870:string)
      n367 = call "Write_Characters_To_File.vi"("file path (dialog if empty)"=w856, "advisory dialog? (display:T)"=w872, "character string"=w870, "append to file? (new file:F)"=w873, "Lock File"=w863) -> ()  [unwired: 4 out]
    }
    frame #17 {
      n368 = case shown="\"Show Setup\"" w885 {
        frame "Show Setup" {
          n369 = Current VI's Path() -> (path=w887:path)
          n370 = call "Open_Close_Front_Panel.ph.vi"("Front Panel Window:Open"=FALSE, "VI path"=w887) -> ()  [unwired: 2 out]
        }
        frame "Take a New Calibration Point", Default {
        }
      }
    }
  }
